vi "bigcryo-T-read.vi"(11 "Lakeshore Address":refnum<visa-resource-name>="COM7") -> (2 "VTI Temp [K]":dbl, 3 "Sample Temp [K]":dbl)   [LabVIEW 2019]
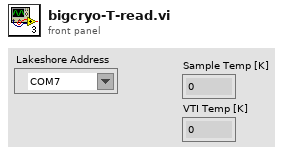
[diagram p1: front panel]
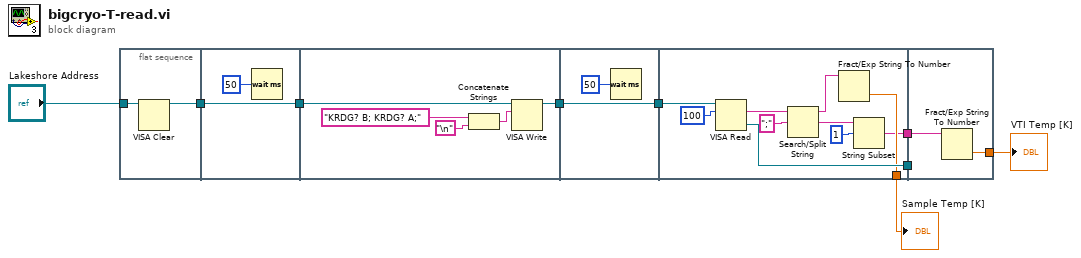
[diagram p0: block diagram]
diagram:
  n1 = flat-sequence {
    tunnel: "Lakeshore Address" -> [w11]
    tunnel: [w10] -> w4
    tunnel: w4 -> [w13]
    tunnel: [w13] -> w3
    tunnel: [w17] -> w9
    tunnel: w3 -> [w18]
    tunnel: w9 -> [w20]
    tunnel: [w20] -> w8
    tunnel: [w29] -> w7
    tunnel: w8 -> [w30]
    tunnel: [w23] -> w2
    tunnel: [w21] -> w1
    tunnel: [w32] -> w5
    tunnel: w7 -> [_]
    tunnel: w1 -> [w31]
    frame #0 {
      n2 = VISA Clear(VISA resource name=w11) -> (VISA resource name out=w10:refnum<visa-resource-name>)  [unwired: 1 in, 1 out]
    }
    frame #1 {
      n3 = Wait (ms)(milliseconds to wait=50) -> ()  [unwired: 1 out]
    }
    frame #2 {
      n4 = Concatenate Strings("KRDG? B; KRDG? A;" ("write buffer"), "\n") -> (w14:string)
      n5 = VISA Write(VISA resource name=w18, write buffer=w14) -> (VISA resource name out=w17:refnum<visa-resource-name>)  [unwired: 1 in, 2 out]
    }
    frame #3 {
      n6 = Wait (ms)(milliseconds to wait=50) -> ()  [unwired: 1 out]
    }
    frame #4 {
      n7 = VISA Read(VISA resource name=w30, byte count=u32 100) -> (VISA resource name out=w29:refnum<visa-resource-name>, read buffer=w22:string)  [unwired: 1 in, 2 out]
      n8 = Search/Split String(string=w22, search string/char (-)=";") -> (substring before match=w24:string, match + rest of string=w26:string)  [unwired: 1 in, 1 out]
      n9 = Fract/Exp String To Number(string=w24) -> (number=w23:dbl)  [unwired: 3 in, 1 out]
      n10 = String Subset(string=w26, offset (0)=u32 1 ("byte count")) -> (substring=w21:string)  [unwired: 1 in]
    }
    frame #5 {
      n11 = Fract/Exp String To Number(string=w31) -> (number=w32:dbl)  [unwired: 3 in, 1 out]
    }
  }
  "Sample Temp [K]" <- w2
  "VTI Temp [K]" <- w5
